vi "_TangoDeviceStateAndStatus.vi"(5 "error in":errorcluster, 6 "Device Name":string) -> (0 "Status":string, 1 "State String":string, 2 "State Color":u32(colorbox)=16448250, 3 "State Code":i16, 4 "error out":errorcluster)   [LabVIEW 2014, in "tango.lvlib"]
uses:
  tango.lvlib
  tango_binding.so
panel:
  out "State/Status":string[](array[string])
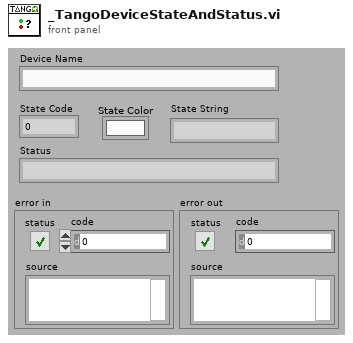
[diagram p1: front panel]
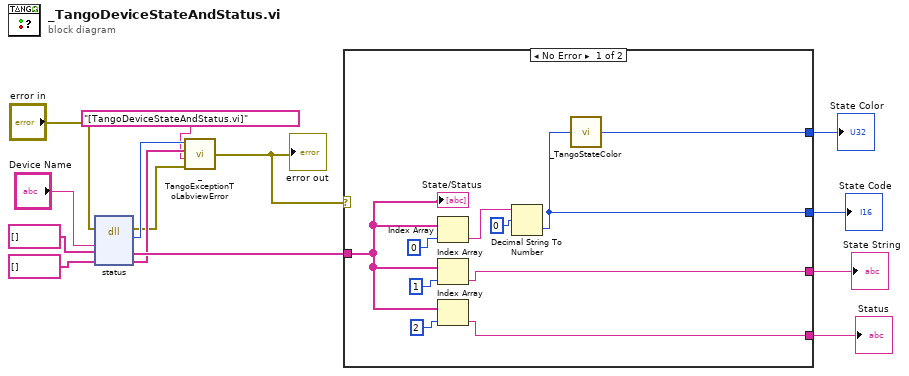
[diagram p0: block diagram]
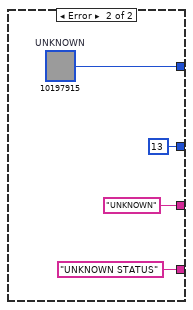
[diagram p2: hidden frame]
diagram:
  n1 = dll-call lib="tango_binding.*" fn="status"(error in="error in", "dev_name"="Device Name", "status"=string[] [] ("State/Status"), "error_stack"=string[] [] ("Error Stack")) -> (error out=w6:errorcluster, w9:i32, "status"=w14:string[], "error_stack"=w8:string[])  [unwired: 3 in, 1 out]
  n2 = call "_TangoExceptionToLabviewError.vi"("error in"=w6, "location"="[TangoDeviceStateAndStatus.vi]", "error stack"=w8, "error code"=w9) -> ("error out"=w5:errorcluster)
  "error out" <- w5
  n3 = case shown="No Error" w5 {
    tunnel: w14 -> [w21 _]
    tunnel: [w15 w28] -> w4
    tunnel: [w18 "UNKNOWN"] -> w3
    tunnel: [w17 "UNKNOWN STATUS"] -> w2
    tunnel: [w16 13] -> w1
    frame No Error {
      n4 = Index Array(array=w21, index=0 ("indice")) -> (element=w20:string)
      n5 = Index Array(array=w21, index=1 ("indice")) -> (element=w18:string)
      n6 = Index Array(array=w21, index=2 ("indice")) -> (element=w17:string)
      n7 = Decimal String To Number(string=w20, offset=0) -> (number=w16:i32)  [unwired: 1 in, 1 out]
      n8 = call "_TangoStateColor.vi"("State"=w16) -> ("State Color"=w15:u32)
      "State/Status" <- w21
    }
    frame Error {
      w28 = u32 10197915  # UNKNOWN
    }
  }
  "State Color" <- w4
  "Status" <- w2
  "State Code" <- w1
  "State String" <- w3
